vi "Performance Test.vi"() -> ()   [LabVIEW 2021]
uses:
  ChannelCommon/typedef/Benchmark Stats.ctl
  ChannelCommon/typedef/Datatype Waveform.ctl
  CIFChannels/Typedef/Direction.ctl
  ChannelCommon/typedef/FIFO Config.ctl
  CIF_NIChn_FIFO_DAQ.lvclass
  D:/dev/Packages/Channel_Manager/src/CIFChannels/CIFChannels.lvclass
  <vilib>/Platform/TimedLoop/XDataNode/timing_clust.ctl
  <vilib>/Platform/TimedLoop/XDataNode/nitl_modes.ctl
  <vilib>/Platform/TimedLoop/XDataNode/wakeup.ctl
  ChannelCommon/typedef/TimeStamps.ctl
  CIFChannels/CIFChannels.lvclass/CIFChannels.ctl
  <vilib>/CIF Foundation/CIF Utilities/Statistics/I64/Stats_I64_CIF_U.lvclass/Stats_I64_CIF_U.ctl
  <vilib>/CIF Foundation/CIF Utilities/DataTypes/Flatten U64.vi
  <vilib>/CIF Foundation/CIF Utilities/Statistics/I64/Get Stats.vi
  <vilib>/Platform/TimedLoop/XDataNode/XDataNode.xnode
  <vilib>/Platform/TimedLoop/XDataNode/XDNodeRunTimeDep.lvlib
  CIFChannels/CIFChannels.lvclass
  ChannelCommon/ChannelCommon.lvlib
panel:
  out "Data Out":T1[](array[typedef])=[{"measurement"=array[200001 elements], "dT"=43.0, "Timestamp"=2, "Read Lock"=FALSE}, {"measurement"=array[200001 elements], "dT"=34.0, "Timestamp"=1, "Read Lock"=FALSE}]
  out "Flatten (us) 2":T2
  out "Write 3":T2={"Max"=465, "Average"=431.350724981784, "Min"=423}
  out "Flatten (us) 3":T2={"Max"=1364, "Average"=894.6544650860508, "Min"=878}
  out "timed out? Inline":bool
  out "Read (us) 2":T2={"Max"=1823, "Average"=1599.4859063832048, "Min"=1467}
  out "Flatten (us) TO":T2
  out "Channel R/W (us) TO":T2={"Max"=45, "Average"=11.444175177596316, "Min"=10}
  out "Flatten (us)":T2
  out "Channel R/W (us)":T2={"Max"=4009, "Average"=3804.247500241507, "Min"=2568}
  out "avg TO":dbl=1.2770776500110515e-05
  out "max TO":dbl=2.531000063754618e-05
  out "timed out?":bool=TRUE
  out "timed out?":bool
  out "avg channel":dbl=0.0037815884919982635
  out "max channel":dbl=0.00401990699901944
  out "pass":bool
  out "error out":errorcluster
  # "Worst case with constant writing.  Timing will be impacted by wait for data to avoid timeout."
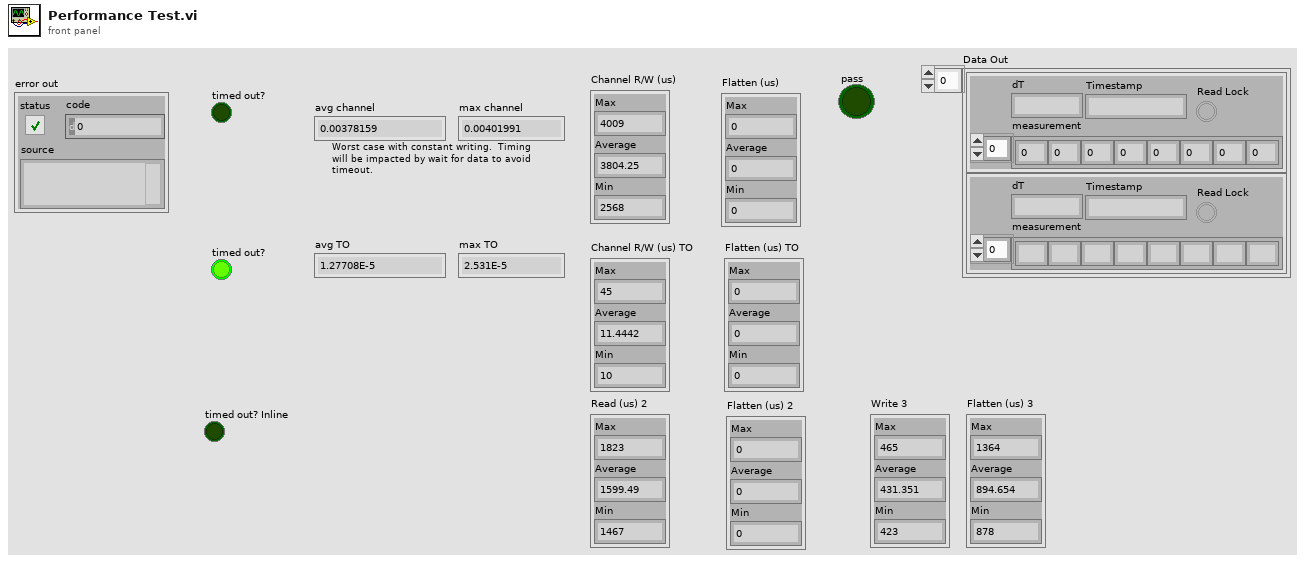
[diagram p1: front panel]
types:
  T1 = typedef "ChannelCommon.lvlib/Datatype Waveform.ctl" = cluster{"measurement":dbl[], "dT":dbl, "Timestamp":i64, "Read Lock":bool}
  T2 = typedef "ChannelCommon.lvlib/Benchmark Stats.ctl" = cluster{"Max":i64, "Average":dbl, "Min":i64}
  T3 = typedef "ChannelCommon.lvlib/FIFO Config.ctl" = cluster{"Max Bytes/Msg":u64, "Max Msg/FIFO":u64, "Flags":u64}
  T4 = typedef "CIFChannels.lvclass/Direction.ctl" = enum16{"Publisher", "Subscriber"}
  T5 = typedef "ChannelCommon.lvlib/TimeStamps.ctl" = cluster{"ClockID":u8, "T0":i64, "T_Out":i64}
  T6 = typedef "XDNodeRunTimeDep.lvlib/timing_clust.ctl" = cluster{"Expected End [f-1]":u64, "Actual End [f-1]":u64, "Finished Late? [f-1]":bool, "Expected End [i-1]":u64, "Actual End [i-1]":u64, "Finished Late? [i-1]":bool, "Expected Start [i]":u64, "Actual Start [i]":u64, "Expected Start [f]":u64, "Actual Start [f]":u64, "Source Name":string, "Structure Name":string, "Period":i64, "Deadline":i64, "Offset":i64, "Start":i64, "Priority":i32, "Timeout":i32, "Mode":T7, "Wakeup Reason":T8, "Error":errorcluster, "Source Type":string, "Secondary Source Type":string, "Global End Time":u64, "Global Start Time":u64, "Frame Duration":u64, "Iteration Duration":u64, "Assigned CPU":i32, "I/O Scan Engine Mode":u32}
  T7 = typedef "XDNodeRunTimeDep.lvlib/nitl_modes.ctl" = enum32{"No Change", "Process missed periods, maintain original phase", "Discard missed periods, maintain original phase", "Process missed periods, ignore original phase", "Discard missed periods, ignore original phase"}
  T8 = typedef "XDNodeRunTimeDep.lvlib/wakeup.ctl" = enum32{"Normal", "Aborted", "Asynchronous wakeup", "Timing source error", "Timed loop error", "Timeout"}
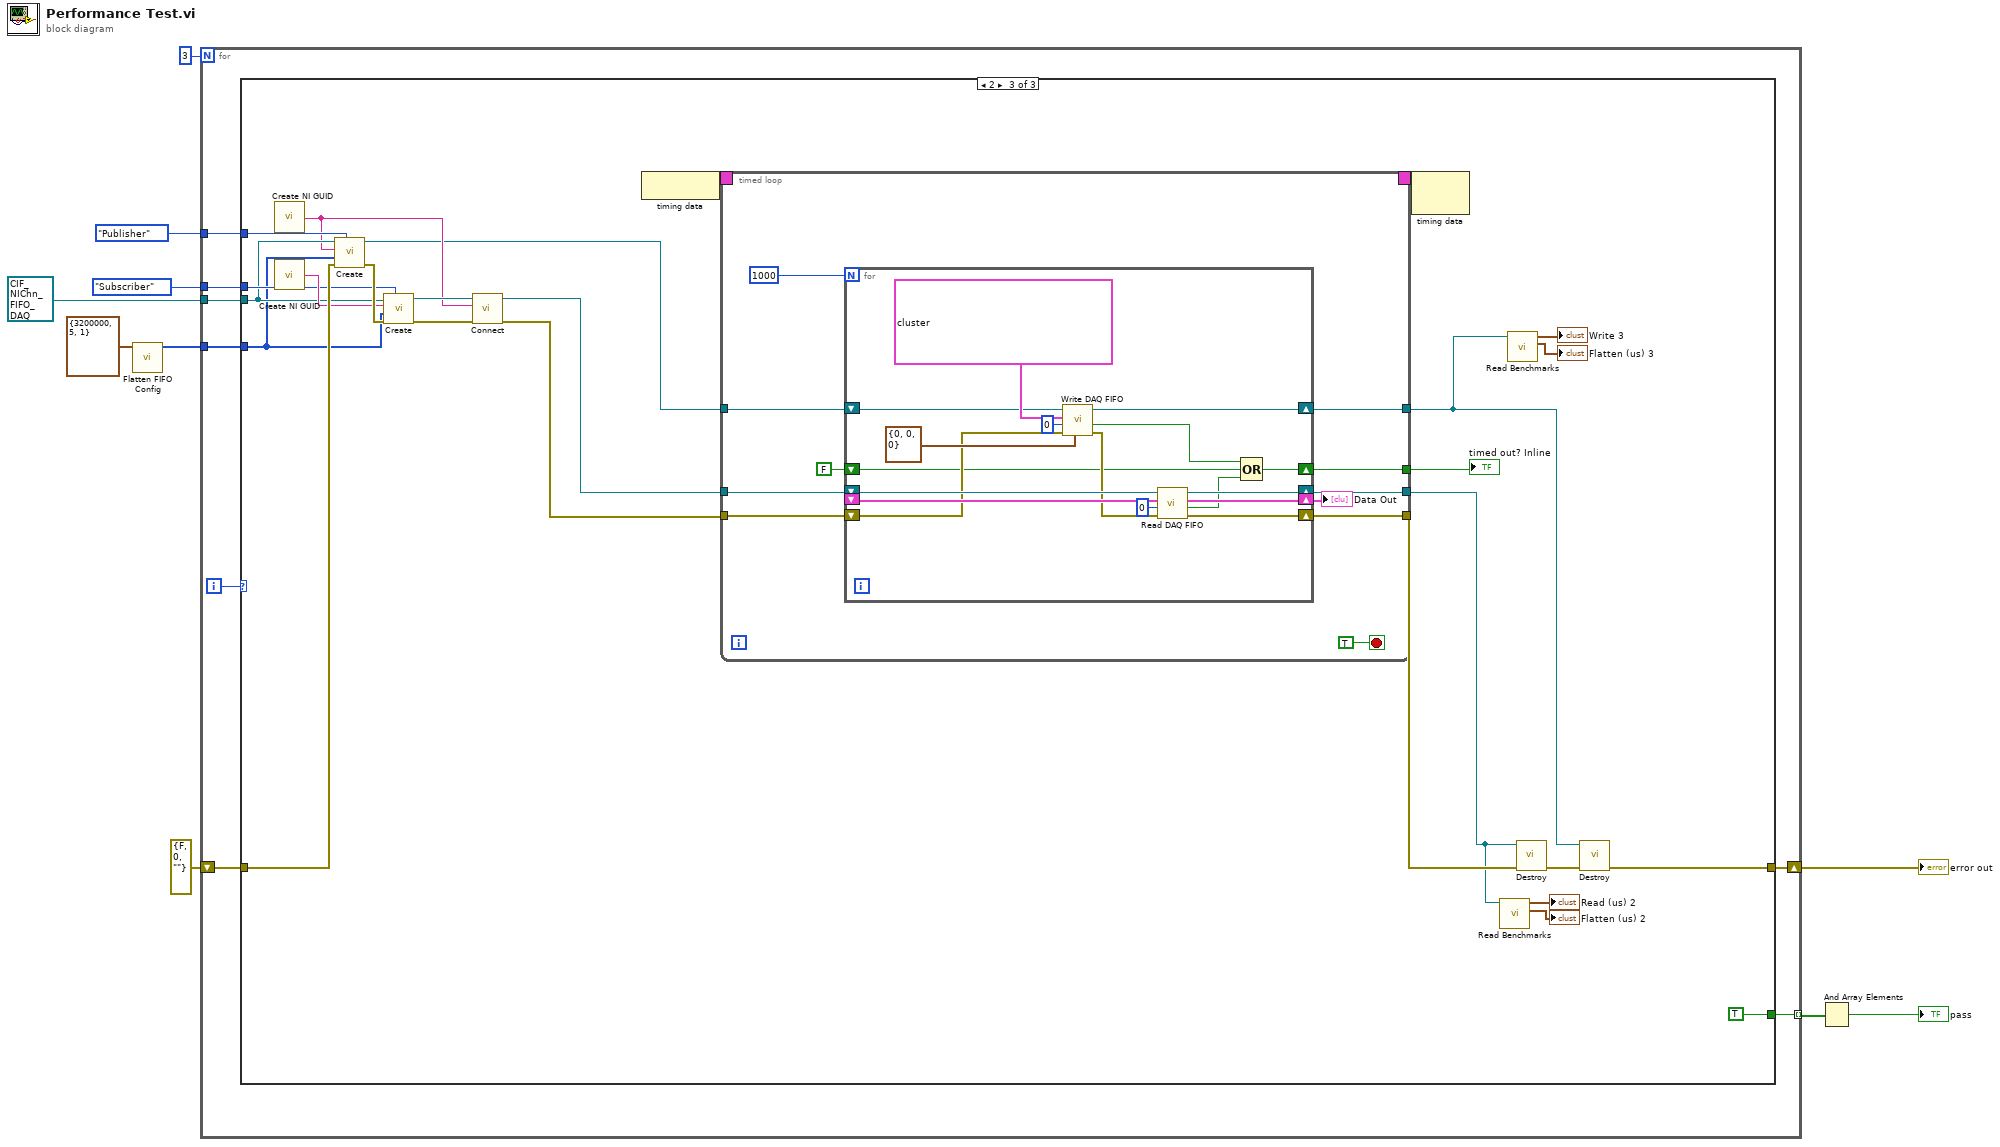
[diagram p0: block diagram]
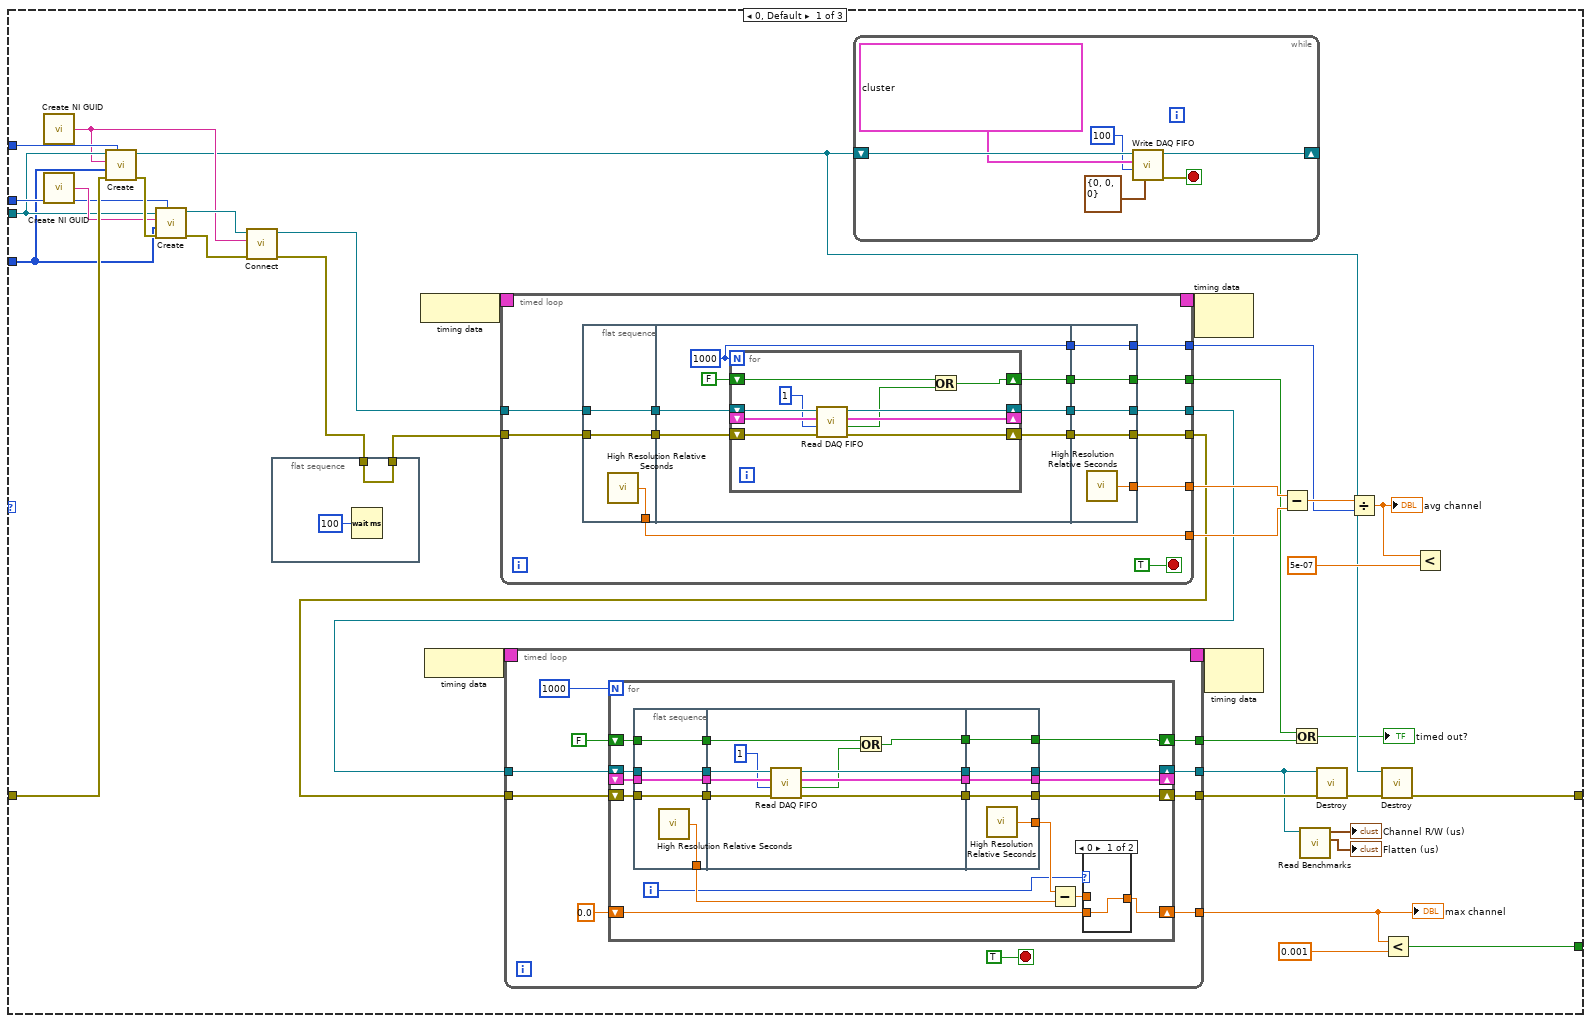
[diagram p2: hidden frame]
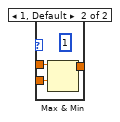
[diagram p3: hidden frame]
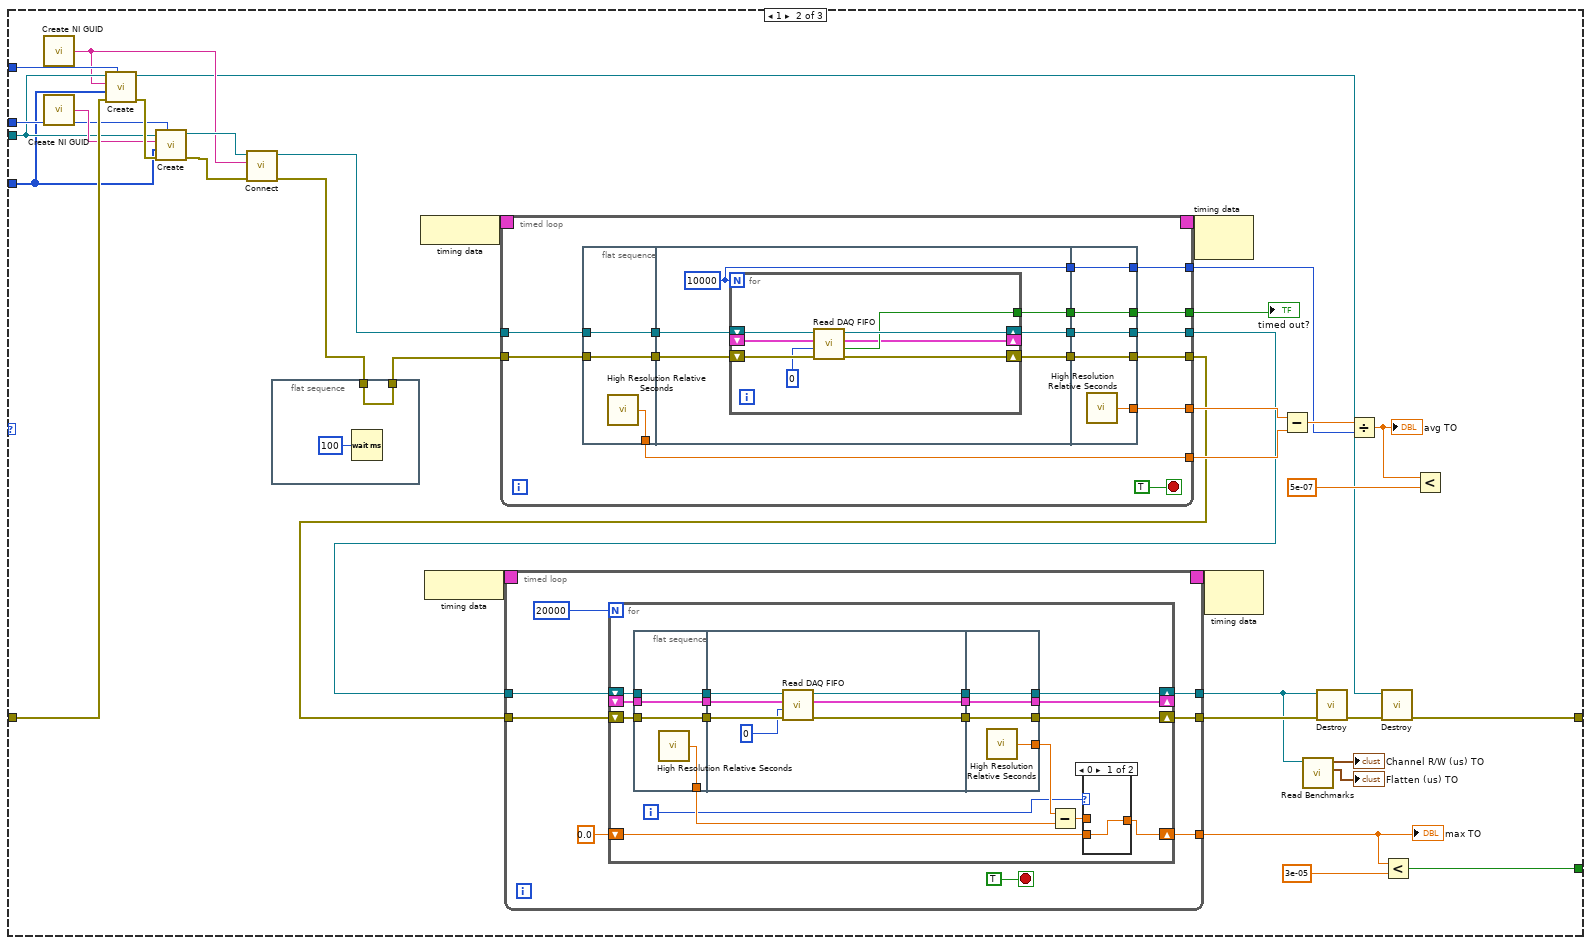
[diagram p4: hidden frame]
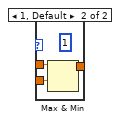
[diagram p5: hidden frame]
diagram:
  n1 = call "Flatten FIFO Config.vi"("FIFO Config in"=T3 {"Max Bytes/Msg"=3200000, "Max Msg/FIFO"=5, "Flags"=1}) -> ("Flattened FIFO Config"=w2:u8[])  [unwired: 10 in]
  n2 = for {
    N: 3 -> [_]
    tunnel: [w18] -> w8 mode=indexing
    shift-right: [w17] -> w10
    shift-left: errorcluster {"status"=FALSE, "code"=0, "source"=""} ("error out") -> [w15]
    tunnel: Direction."Publisher" ("Direction") -> [w14]
    tunnel: Direction."Subscriber" ("Direction") -> [w13]
    tunnel: refnum<class "CIF_NIChn_FIFO_DAQ.lvclass"> refnum ("CIF_NIChn_FIFO_DAQ.lvclass") -> [w12]
    tunnel: w2 -> [w11]
    i -> [w16]
    n3 = case shown="2" w16 {
      tunnel: [w42 w190 TRUE] -> w18
      tunnel: [w27 w175 w308] -> w17
      tunnel: w15 -> [w40 w188 w319]
      tunnel: w14 -> [w38 w186 w317]
      tunnel: w13 -> [w37 w185 w316]
      tunnel: w12 -> [w36 w184 w315]
      tunnel: w11 -> [w32 w180 w311]
      frame 0, Default {
        n4 = call <vilib>:"Create NI GUID.vi"() -> ("NI GUID"=w34:string)
        n5 = call <vilib>:"Create NI GUID.vi"() -> ("NI GUID"=w39:string)
        n6 = call-dynamic "Create.vi"("Direction"=w38, "error in (no error)"=w40, "Custom Config Data"=w32, "Name"=w34, "CIFFIFO in"=w36) -> ("error out"=w41:errorcluster, "CIFFIFO out"=w28:refnum<class "CIF_NIChn_FIFO_DAQ.lvclass">)  [unwired: 5 in]
        n7 = call-dynamic "Create.vi"("Direction"=w37, "error in (no error)"=w41, "Custom Config Data"=w32, "Name"=w39, "CIFFIFO in"=w36) -> ("error out"=w33:errorcluster, "CIFFIFO out"=w35:refnum<class "CIF_NIChn_FIFO_DAQ.lvclass">)  [unwired: 5 in]
        n8 = call-dynamic "Connect.vi"("error in (no error)"=w33, "Connection Name"=w34, "CIFTag in"=w35) -> ("error out"=w26:errorcluster, "CIFTag out"=w31:refnum<class "CIF_NIChn_FIFO_DAQ.lvclass">)  [unwired: 7 in]
        n9 = flat-sequence {
          tunnel: w26 -> [w58]
          tunnel: [w58] -> w25
          frame #0 {
            n10 = Wait (ms)(milliseconds to wait=u32 100) -> ()  [unwired: 1 out]
          }
        }
        n11 = node-c288() -> (w56:T6)
        n12 = node-c288() -> (w54:T6)
        n13 = timed-loop {
          timing: w56 -> [_]
          timing-out: [_] -> w55
          tunnel: w31 -> [w139]
          tunnel: w25 -> [w138]
          tunnel: [w134] -> w48
          tunnel: [w132] -> w47
          tunnel: [w130] -> w52
          tunnel: [w129] -> w51
          tunnel: [w128] -> w49
          tunnel: [w126] -> w20
          stop <- TRUE stop-if-true
          n14 = flat-sequence {
            tunnel: w138 -> [w141]
            tunnel: w139 -> [w142]
            tunnel: [w142] -> w136
            tunnel: [w141] -> w135
            tunnel: [w140] -> w129
            tunnel: w136 -> [w149]
            tunnel: w135 -> [w148]
            tunnel: [w147] -> w133
            tunnel: [w146] -> w131
            tunnel: [w145] -> w127
            tunnel: [w143] -> w125
            tunnel: [w164] -> w134
            tunnel: w133 -> [w164]
            tunnel: [w163] -> w132
            tunnel: w131 -> [w163]
            tunnel: [w162] -> w130
            tunnel: [w161] -> w128
            tunnel: w127 -> [w161]
            tunnel: [w160] -> w126
            tunnel: w125 -> [w160]
            frame #0 {
              n15 = call <vilib>:"High Resolution Relative Seconds.vi"() -> ("relative seconds"=w140:dbl)
            }
            frame #1 {
              w145 = 1000
              n16 = for {
                N: w145 -> [_]
                shift-right: [w154] -> w147
                shift-left: w149 -> [w159]
                shift-right: [w157] -> w146
                shift-left: w148 -> [w158]
                shift-right: [w156] -> _
                shift-left: _ -> [w155]
                shift-right: [w150] -> w143
                shift-left: FALSE -> [w152]
                n17 = call-dynamic "Read DAQ FIFO.vi"("error in (no error)"=w158, "Timeout (ms)"=1, "Data In"=w155, "CIF_NIChn_FIFO_DAQ in"=w159) -> ("error out"=w157:errorcluster, "timed out?"=w151:bool, "Data Out"=w156:T1[], "CIF_NIChn_FIFO_DAQ out"=w154:refnum<class "CIF_NIChn_FIFO_DAQ.lvclass">)  [unwired: 3 in, 1 out]
                n18 = Or(x=w152, y=w151) -> (x .or. y?=w150:bool)
              }
            }
            frame #2 {
              n19 = call <vilib>:"High Resolution Relative Seconds.vi"() -> ("relative seconds"=w162:dbl)
            }
          }
        }
        n20 = timed-loop {
          timing: w54 -> [_]
          timing-out: [_] -> w53
          tunnel: w48 -> [w74]
          tunnel: w47 -> [w73]
          tunnel: [w71] -> w24
          tunnel: [w70] -> w30
          tunnel: [w67] -> w44
          tunnel: [w65] -> w19
          stop <- TRUE stop-if-true
          n21 = for {
            N: 1000 -> [_]
            shift-right: [w90] -> w71
            shift-left: w74 -> [w92]
            shift-right: [w89] -> w70
            shift-left: w73 -> [w91]
            shift-right: [w83] -> w67
            shift-left: 0.0 -> [w84]
            shift-right: [w82] -> _
            shift-left: _ -> [w88]
            shift-right: [w76] -> w65
            shift-left: FALSE -> [w77]
            i -> [w80]
            n22 = flat-sequence {
              tunnel: w91 -> [w104]
              tunnel: w92 -> [w105]
              tunnel: [w105] -> w96
              tunnel: [w104] -> w95
              tunnel: [w103] -> w86
              tunnel: w88 -> [w102]
              tunnel: [w102] -> w94
              tunnel: [w101] -> w78
              tunnel: w77 -> [w101]
              tunnel: w96 -> [w115]
              tunnel: w95 -> [w114]
              tunnel: [w111] -> w93
              tunnel: w94 -> [w110]
              tunnel: [w112] -> w81
              tunnel: [w113] -> w79
              tunnel: w78 -> [w108]
              tunnel: [w106] -> w75
              tunnel: [w120] -> w90
              tunnel: w93 -> [w120]
              tunnel: [w119] -> w89
              tunnel: [w118] -> w87
              tunnel: [w117] -> w82
              tunnel: w81 -> [w117]
              tunnel: w79 -> [w119]
              tunnel: [w116] -> w76
              tunnel: w75 -> [w116]
              frame #0 {
                n23 = call <vilib>:"High Resolution Relative Seconds.vi"() -> ("relative seconds"=w103:dbl)
              }
              frame #1 {
                n24 = call-dynamic "Read DAQ FIFO.vi"("error in (no error)"=w114, "Timeout (ms)"=1, "Data In"=w110, "CIF_NIChn_FIFO_DAQ in"=w115) -> ("error out"=w113:errorcluster, "timed out?"=w107:bool, "Data Out"=w112:T1[], "CIF_NIChn_FIFO_DAQ out"=w111:refnum<class "CIF_NIChn_FIFO_DAQ.lvclass">)  [unwired: 3 in, 1 out]
                n25 = Or(x=w108, y=w107) -> (x .or. y?=w106:bool)
              }
              frame #2 {
                n26 = call <vilib>:"High Resolution Relative Seconds.vi"() -> ("relative seconds"=w118:dbl)
              }
            }
            n27 = Subtract(x=w87, y=w86) -> (x-y=w85:dbl)
            n28 = case shown="0" w80 {
              tunnel: w85 -> [_ w100]
              tunnel: w84 -> [w97 w99]
              tunnel: [w97 w98] -> w83
              frame 0 {
              }
              frame 1, Default {
                (unwired) u32 1 ("milliseconds to wait")
                n29 = Max & Min(x=w100, y=w99) -> (max(x,y)=w98:dbl)  [unwired: 1 out]
              }
            }
          }
        }
        "max channel" <- w44
        n30 = while {
          shift-right: [w61] -> _
          shift-left: w28 -> [w64]
          stop <- w62 stop-if-true
          n31 = call-dynamic "Write DAQ FIFO.vi"("FIFO Timestamps"=T5 {"ClockID"=0, "T0"=0, "T_Out"=0}, "Timeout (ms)"=100, "Data In"=T1[] [{"measurement"=array[200001 elements], "dT"=43.0, "Timestamp"=2, "Read Lock"=FALSE}, {"measurement"=array[200001 elements], "dT"=34.0, "Timestamp"=1, "Read Lock"=FALSE}] ("DAQ In"), "CIF_NIChn_FIFO_DAQ in"=w64) -> ("error out"=w62:errorcluster, "CIF_NIChn_FIFO_DAQ out"=w61:refnum<class "CIF_NIChn_FIFO_DAQ.lvclass">)  [unwired: 4 in, 2 out]
        }
        n32 = node-c288(w55) -> ()  [unwired: 1 out]
        n33 = node-c288(w53) -> ()  [unwired: 1 out]
        n34 = Subtract(x=w52, y=w51) -> (x-y=w50:dbl)
        n35 = Or(x=w20, y=w19) -> (x .or. y?=→"timed out?":bool)
        n36 = call "Read Benchmarks.vi"("CIFChannels in"=w24) -> ("Flatten (us)"=→"Flatten (us)":T2, "Channel R/W (us)"=→"Channel R/W (us)":T2)  [unwired: 9 in]
        n37 = call-dynamic "Destroy.vi"("error in (no error)"=w30, "CIFFIFO in"=w24) -> ("error out"=w29:errorcluster)  [unwired: 8 in, 1 out]
        n38 = Divide(x=w50, y=w49) -> (x/y=w46:dbl)
        "avg channel" <- w46
        n39 = call-dynamic "Destroy.vi"("error in (no error)"=w29, "CIFFIFO in"=w28) -> ("error out"=w27:errorcluster)  [unwired: 8 in, 1 out]
        n40 = Less?(x=w44, y=0.001) -> (x < y?=w42:bool)
        n41 = Less?(x=w46, y=5e-07) -> ()  [unwired: 1 out]
      }
      frame 1 {
        n42 = call <vilib>:"Create NI GUID.vi"() -> ("NI GUID"=w182:string)
        n43 = call <vilib>:"Create NI GUID.vi"() -> ("NI GUID"=w187:string)
        n44 = call-dynamic "Create.vi"("Direction"=w186, "error in (no error)"=w188, "Custom Config Data"=w180, "Name"=w182, "CIFFIFO in"=w184) -> ("error out"=w189:errorcluster, "CIFFIFO out"=w176:refnum<class "CIF_NIChn_FIFO_DAQ.lvclass">)  [unwired: 5 in]
        n45 = call-dynamic "Create.vi"("Direction"=w185, "error in (no error)"=w189, "Custom Config Data"=w180, "Name"=w187, "CIFFIFO in"=w184) -> ("error out"=w181:errorcluster, "CIFFIFO out"=w183:refnum<class "CIF_NIChn_FIFO_DAQ.lvclass">)  [unwired: 5 in]
        n46 = call-dynamic "Connect.vi"("error in (no error)"=w181, "Connection Name"=w182, "CIFTag in"=w183) -> ("error out"=w174:errorcluster, "CIFTag out"=w179:refnum<class "CIF_NIChn_FIFO_DAQ.lvclass">)  [unwired: 7 in]
        n47 = flat-sequence {
          tunnel: w174 -> [w206]
          tunnel: [w206] -> w173
          frame #0 {
            n48 = Wait (ms)(milliseconds to wait=u32 100) -> ()  [unwired: 1 out]
          }
        }
        n49 = node-c288() -> (w204:T6)
        n50 = node-c288() -> (w202:T6)
        n51 = timed-loop {
          timing: w204 -> [_]
          timing-out: [_] -> w203
          tunnel: w179 -> [w270]
          tunnel: w173 -> [w269]
          tunnel: [w265] -> w196
          tunnel: [w263] -> w195
          tunnel: [w261] -> w200
          tunnel: [w260] -> w199
          tunnel: [w259] -> w197
          tunnel: [w257] -> w172
          stop <- TRUE stop-if-true
          n52 = flat-sequence {
            tunnel: w269 -> [w272]
            tunnel: w270 -> [w273]
            tunnel: [w273] -> w267
            tunnel: [w272] -> w266
            tunnel: [w271] -> w260
            tunnel: w267 -> [w279]
            tunnel: w266 -> [w278]
            tunnel: [w277] -> w264
            tunnel: [w276] -> w262
            tunnel: [w275] -> w258
            tunnel: [w274] -> w256
            tunnel: [w292] -> w265
            tunnel: w264 -> [w292]
            tunnel: [w291] -> w263
            tunnel: w262 -> [w291]
            tunnel: [w290] -> w261
            tunnel: [w289] -> w259
            tunnel: w258 -> [w289]
            tunnel: [w288] -> w257
            tunnel: w256 -> [w288]
            frame #0 {
              n53 = call <vilib>:"High Resolution Relative Seconds.vi"() -> ("relative seconds"=w271:dbl)
            }
            frame #1 {
              w275 = 10000
              n54 = for {
                N: w275 -> [_]
                shift-right: [w284] -> w277
                shift-left: w279 -> [w287]
                shift-right: [w285] -> w276
                shift-left: w278 -> [w286]
                shift-right: [w282] -> _
                shift-left: _ -> [w281]
                tunnel: [w283] -> w274
                n55 = call-dynamic "Read DAQ FIFO.vi"("error in (no error)"=w286, "Timeout (ms)"=0, "Data In"=w281, "CIF_NIChn_FIFO_DAQ in"=w287) -> ("error out"=w285:errorcluster, "timed out?"=w283:bool, "Data Out"=w282:T1[], "CIF_NIChn_FIFO_DAQ out"=w284:refnum<class "CIF_NIChn_FIFO_DAQ.lvclass">)  [unwired: 3 in, 1 out]
              }
            }
            frame #2 {
              n56 = call <vilib>:"High Resolution Relative Seconds.vi"() -> ("relative seconds"=w290:dbl)
            }
          }
        }
        "timed out?" <- w172
        n57 = timed-loop {
          timing: w202 -> [_]
          timing-out: [_] -> w201
          tunnel: w196 -> [w214]
          tunnel: w195 -> [w213]
          tunnel: [w211] -> w169
          tunnel: [w210] -> w178
          tunnel: [w207] -> w192
          stop <- TRUE stop-if-true
          n58 = for {
            N: 20000 -> [_]
            shift-right: [w226] -> w211
            shift-left: w214 -> [w228]
            shift-right: [w225] -> w210
            shift-left: w213 -> [w227]
            shift-right: [w219] -> w207
            shift-left: 0.0 -> [w220]
            shift-right: [w218] -> _
            shift-left: _ -> [w224]
            i -> [w216]
            n59 = flat-sequence {
              tunnel: w227 -> [w239]
              tunnel: w228 -> [w240]
              tunnel: [w240] -> w232
              tunnel: [w239] -> w231
              tunnel: [w238] -> w222
              tunnel: w224 -> [w237]
              tunnel: [w237] -> w230
              tunnel: w232 -> [w247]
              tunnel: w231 -> [w243]
              tunnel: [w246] -> w229
              tunnel: w230 -> [w244]
              tunnel: [w245] -> w217
              tunnel: [w242] -> w215
              tunnel: [w251] -> w226
              tunnel: w229 -> [w251]
              tunnel: [w250] -> w225
              tunnel: [w249] -> w223
              tunnel: [w248] -> w218
              tunnel: w217 -> [w248]
              tunnel: w215 -> [w250]
              frame #0 {
                n60 = call <vilib>:"High Resolution Relative Seconds.vi"() -> ("relative seconds"=w238:dbl)
              }
              frame #1 {
                n61 = call-dynamic "Read DAQ FIFO.vi"("error in (no error)"=w243, "Timeout (ms)"=0, "Data In"=w244, "CIF_NIChn_FIFO_DAQ in"=w247) -> ("error out"=w242:errorcluster, "Data Out"=w245:T1[], "CIF_NIChn_FIFO_DAQ out"=w246:refnum<class "CIF_NIChn_FIFO_DAQ.lvclass">)  [unwired: 3 in, 2 out]
              }
              frame #2 {
                n62 = call <vilib>:"High Resolution Relative Seconds.vi"() -> ("relative seconds"=w249:dbl)
              }
            }
            n63 = Subtract(x=w223, y=w222) -> (x-y=w221:dbl)
            n64 = case shown="0" w216 {
              tunnel: w221 -> [_ w236]
              tunnel: w220 -> [w233 w235]
              tunnel: [w233 w234] -> w219
              frame 0 {
              }
              frame 1, Default {
                (unwired) u32 1 ("milliseconds to wait")
                n65 = Max & Min(x=w236, y=w235) -> (max(x,y)=w234:dbl)  [unwired: 1 out]
              }
            }
          }
        }
        "max TO" <- w192
        n66 = node-c288(w203) -> ()  [unwired: 1 out]
        n67 = node-c288(w201) -> ()  [unwired: 1 out]
        n68 = Subtract(x=w200, y=w199) -> (x-y=w198:dbl)
        n69 = call "Read Benchmarks.vi"("CIFChannels in"=w169) -> ("Flatten (us)"=→"Flatten (us) TO":T2, "Channel R/W (us)"=→"Channel R/W (us) TO":T2)  [unwired: 9 in]
        n70 = call-dynamic "Destroy.vi"("error in (no error)"=w178, "CIFFIFO in"=w169) -> ("error out"=w177:errorcluster)  [unwired: 8 in, 1 out]
        n71 = Divide(x=w198, y=w197) -> (x/y=w194:dbl)
        "avg TO" <- w194
        n72 = call-dynamic "Destroy.vi"("error in (no error)"=w177, "CIFFIFO in"=w176) -> ("error out"=w175:errorcluster)  [unwired: 8 in, 1 out]
        n73 = Less?(x=w192, y=3e-05) -> (x < y?=w190:bool)
        n74 = Less?(x=w194, y=5e-07) -> ()  [unwired: 1 out]
      }
      frame 2 {
        n75 = call <vilib>:"Create NI GUID.vi"() -> ("NI GUID"=w313:string)
        n76 = call <vilib>:"Create NI GUID.vi"() -> ("NI GUID"=w318:string)
        n77 = call-dynamic "Create.vi"("Direction"=w317, "error in (no error)"=w319, "Custom Config Data"=w311, "Name"=w313, "CIFFIFO in"=w315) -> ("error out"=w320:errorcluster, "CIFFIFO out"=w305:refnum<class "CIF_NIChn_FIFO_DAQ.lvclass">)  [unwired: 5 in]
        n78 = call-dynamic "Create.vi"("Direction"=w316, "error in (no error)"=w320, "Custom Config Data"=w311, "Name"=w318, "CIFFIFO in"=w315) -> ("error out"=w312:errorcluster, "CIFFIFO out"=w314:refnum<class "CIF_NIChn_FIFO_DAQ.lvclass">)  [unwired: 5 in]
        n79 = call-dynamic "Connect.vi"("error in (no error)"=w312, "Connection Name"=w313, "CIFTag in"=w314) -> ("error out"=w302:errorcluster, "CIFTag out"=w310:refnum<class "CIF_NIChn_FIFO_DAQ.lvclass">)  [unwired: 7 in]
        n80 = node-c288() -> (w322:T6)
        n81 = timed-loop {
          timing: w322 -> [_]
          timing-out: [_] -> w321
          tunnel: w310 -> [w333]
          tunnel: w302 -> [w332]
          tunnel: [w330] -> w303
          tunnel: [w329] -> w304
          tunnel: [w324] -> w307
          tunnel: w305 -> [w327]
          tunnel: [w326] -> w298
          stop <- TRUE stop-if-true
          n82 = for {
            N: 1000 -> [_]
            shift-right: [w346] -> w330
            shift-left: w333 -> [w350]
            shift-right: [w349] -> w329
            shift-left: w332 -> [w343]
            shift-right: [w348] -> w323
            shift-left: _ -> [w347]
            shift-right: [w340] -> w326
            shift-left: w327 -> [w341]
            shift-right: [w335] -> w324
            shift-left: FALSE -> [w336]
            n83 = call-dynamic "Write DAQ FIFO.vi"("FIFO Timestamps"=T5 {"ClockID"=0, "T0"=0, "T_Out"=0}, "error in (no error)"=w343, "Timeout (ms)"=0, "Data In"=T1[] [{"measurement"=array[200001 elements], "dT"=43.0, "Timestamp"=2, "Read Lock"=FALSE}, {"measurement"=array[200001 elements], "dT"=34.0, "Timestamp"=1, "Read Lock"=FALSE}] ("DAQ In"), "CIF_NIChn_FIFO_DAQ in"=w341) -> ("error out"=w342:errorcluster, "timed out?"=w334:bool, "CIF_NIChn_FIFO_DAQ out"=w340:refnum<class "CIF_NIChn_FIFO_DAQ.lvclass">)  [unwired: 3 in, 1 out]
            n84 = call-dynamic "Read DAQ FIFO.vi"("error in (no error)"=w342, "Timeout (ms)"=0, "Data In"=w347, "CIF_NIChn_FIFO_DAQ in"=w350) -> ("error out"=w349:errorcluster, "timed out?"=w337:bool, "Data Out"=w348:T1[], "CIF_NIChn_FIFO_DAQ out"=w346:refnum<class "CIF_NIChn_FIFO_DAQ.lvclass">)  [unwired: 3 in, 1 out]
            n85 = Compound Arithmetic op=OR(w334, w336, w337) -> (w335:bool)
          }
          "Data Out" <- w323
        }
        "timed out? Inline" <- w307
        n86 = node-c288(w321) -> ()  [unwired: 1 out]
        n87 = call "Read Benchmarks.vi"("CIFChannels in"=w303) -> ("Flatten (us)"=→"Flatten (us) 2":T2, "Channel R/W (us)"=→"Read (us) 2":T2)  [unwired: 9 in]
        n88 = call "Read Benchmarks.vi"("CIFChannels in"=w298) -> ("Flatten (us)"=→"Flatten (us) 3":T2, "Channel R/W (us)"=→"Write 3":T2)  [unwired: 9 in]
        n89 = call-dynamic "Destroy.vi"("error in (no error)"=w304, "CIFFIFO in"=w303) -> ("error out"=w309:errorcluster)  [unwired: 8 in, 1 out]
        n90 = call-dynamic "Destroy.vi"("error in (no error)"=w309, "CIFFIFO in"=w298) -> ("error out"=w308:errorcluster)  [unwired: 8 in, 1 out]
      }
    }
  }
  "error out" <- w10
  n91 = And Array Elements(Boolean array=w8) -> (logical AND=→"pass":bool)
